vi "Create.vi"(9 "jettl":refnum<class "jettl.lvclass">, 10 "Self Alias":string, 11 "Base Event in":refnum<class "Base Event.lvclass">) -> (3 "Base Event out":refnum<class "Base Event.lvclass">)   [LabVIEW 2021, in "jettl.lvlib" / "Base Event.lvlib" / "Base Event.lvclass"]
uses:
  Base Event.lvclass
  Base Event.lvclass/Base Event.ctl
  Error/Error.lvlib
  Msg Strategy/Msg Strategy.lvclass
  Addresses Strategy/Addresses Strategy/Addresses Strategy.lvclass
  jettl/jettl.lvclass
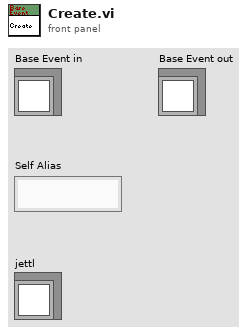
[diagram p1: front panel]
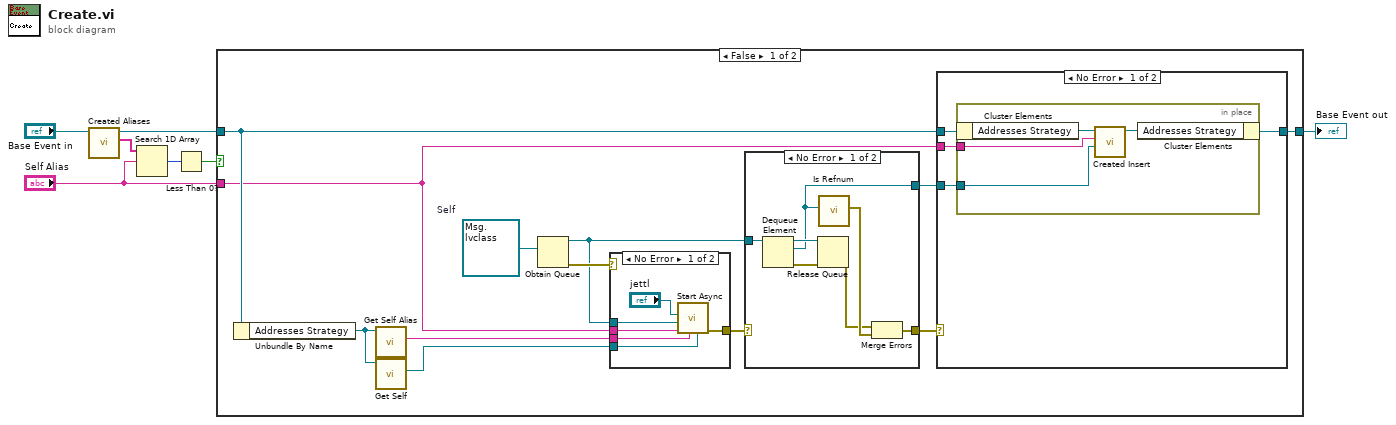
[diagram p0: block diagram]
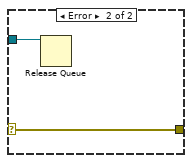
[diagram p2: hidden frame]
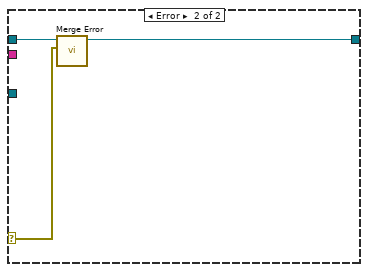
[diagram p4: hidden frame]
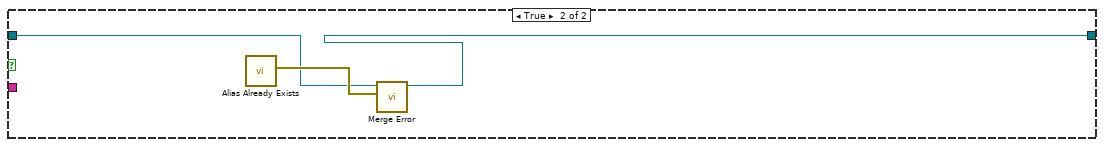
[diagram p5: hidden frame]
diagram:
  n1 = call-dynamic "Created Aliases.vi"("Base Event in"="Base Event in") -> ("Created Aliases"=w4:string[], "Base Event out"=w5:refnum<class "Base Event.lvclass">)  [unwired: 9 in]
  n2 = Search 1D Array(1D array=w4, element="Self Alias") -> (index of element=w2:i32)  [unwired: 1 in]
  n3 = Less Than 0?(x=w2) -> (x < 0?=w1:bool)
  n4 = case shown="False" w1 {
    tunnel: w5 -> [w14 w48]
    tunnel: "Self Alias" -> [w8 _]
    tunnel: [w19 w47] -> w7
    frame False {
      w10 = refnum<user-event> refnum  # Self
      n5 = Unbundle By Name(w14) -> ("Addresses Strategy"=w13:refnum<class "Addresses Strategy.lvclass">)
      n6 = call-dynamic "Get Self Alias.vi"("Addresses Strategy in"=w13) -> ("Self Alias"=w11:string)  [unwired: 10 in]
      n7 = call-dynamic "Get Self.vi"("Addresses Strategy in"=w13) -> ("Self"=w12:refnum<user-event>)  [unwired: 10 in]
      n8 = Obtain Queue(element data type=w10) -> (queue out=w9:refnum<queue>, error out=w18:errorcluster)  [unwired: 4 in, 1 out]
      n9 = case shown="No Error" w18 {
        selector: w18 -> [_ w35]
        tunnel: [w34 w35] -> w16
        tunnel: w8 -> [w31 _]
        tunnel: w12 -> [w33 _]
        tunnel: w11 -> [w32 _]
        tunnel: w9 -> [w30 _]
        frame No Error {
          n10 = call "Start Async.vi"("Creator"=w33, "Creator Alias"=w32, "Self Alias"=w31, "Queue of Self"=w30, "jettl"="jettl") -> ("error out"=w34:errorcluster)  [unwired: 6 in]
        }
        frame Error {
        }
      }
      n11 = case shown="No Error" w16 {
        selector: w16 -> [_ w28]
        tunnel: [w24 w28] -> w17
        tunnel: w9 -> [w21 w27]
        tunnel: [w20 _] -> w15
        frame No Error {
          n12 = Dequeue Element(queue=w21) -> (queue out=w25:refnum<queue>, element=w20:refnum<user-event>, error out=w26:errorcluster)  [unwired: 2 in, 1 out]
          n13 = Release Queue(queue=w25, error in (no error)=w26) -> (error out=w22:errorcluster)  [unwired: 1 in, 2 out]
          n14 = call "Is Refnum.vi"("Self"=w20) -> ("Error"=w23:errorcluster)  [unwired: 10 in]
          n15 = Merge Errors(w22, w23) -> (w24:errorcluster)
        }
        frame Error {
          n16 = Release Queue(queue=w27) -> ()  [unwired: 2 in, 3 out]
        }
      }
      n17 = case shown="No Error" w17 {
        selector: w17 -> [_ w46]
        tunnel: w14 -> [w37 w45]
        tunnel: [w36 w44] -> w19
        tunnel: w15 -> [w39 _]
        tunnel: w8 -> [w38 _]
        frame No Error {
          n18 = in-place {
            in-place-border: w39 -> [w40]
            in-place-border: w38 -> [w41]
            n19 = in-place-cluster #1(w37) -> ("Addresses Strategy"=w43:refnum<class "Addresses Strategy.lvclass">)
            n20 = call-dynamic "Created Insert.vi"("Created"=w40, "Created Alias"=w41, "Addresses Strategy in"=w43) -> ("Addresses Strategy out"=w42:refnum<class "Addresses Strategy.lvclass">)  [unwired: 8 in]
            n21 = in-place-cluster #1("Addresses Strategy"=w42) -> (w36:refnum<class "Base Event.lvclass">)
          }
        }
        frame Error {
          n22 = call-dynamic "Merge Error.vi"("Error"=w46, "Base Event in"=w45) -> ("Base Event out"=w44:refnum<class "Base Event.lvclass">)  [unwired: 9 in]
        }
      }
    }
    frame True {
      n23 = call "Alias Already Exists.vi"() -> ("Error"=w49:errorcluster)  [unwired: 11 in]
      n24 = call-dynamic "Merge Error.vi"("Error"=w49, "Base Event in"=w48) -> ("Base Event out"=w47:refnum<class "Base Event.lvclass">)  [unwired: 9 in]
    }
  }
  "Base Event out" <- w7
